vi "Wave-Read EPL Chunk.vi"(0 "Wave File":path, 11 "error in (no error)":errorcluster) -> (8 "EPL Variables":T1[](array[typedef]), 15 "error out":errorcluster)   [LabVIEW 2020]
uses:
  Wave-EPL Chunk Variable.ctl
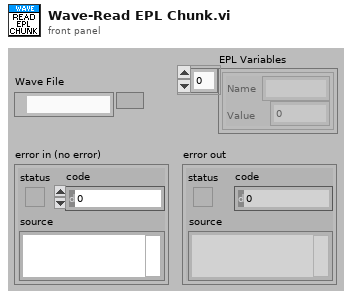
[diagram p1: front panel]
types:
  T1 = typedef "Wave-EPL Chunk Variable.ctl" = cluster{"Name":string, "Value":dbl}
  T2 = typedef "Wave-Chunk Info.ctl" = cluster{"ID":string, "Size":u32}
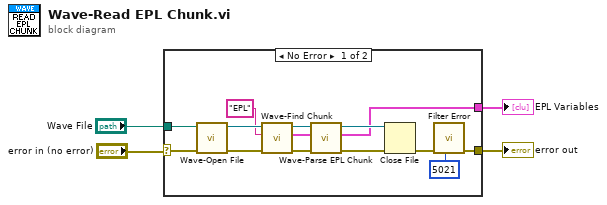
[diagram p0: block diagram]
diagram:
  n1 = case shown="No Error" "error in (no error)" {
    selector: "error in (no error)" -> [w16 w19]
    tunnel: [w6 w19] -> w3
    tunnel: "Wave File" -> [w18 _]
    tunnel: [w7 _] -> w1
    frame No Error {
      n2 = call "Wave-Open File.vi"("error in (no error)"=w16, "Path"=w18) -> ("error out"=w17:errorcluster, "refnum out"=w14:refnum<file>)  [unwired: 8 in]
      n3 = call "Wave-Find Chunk.vi"("error in (no error)"=w17, "Chunk ID"="EPL", "Refnum"=w14) -> ("error out"=w12:errorcluster, "chunk info"=w10:T2, "refnum out"=w11:refnum<file>)  [unwired: 6 in]
      n4 = call "Wave-Parse EPL Chunk.vi"("error in (no error)"=w12, "chunk info"=w10, "refnum"=w11) -> ("error out"=w9:errorcluster, "EPL Variables"=w7:T1[], "refnum out"=w8:refnum<file>)  [unwired: 6 in]
      n5 = Close File(refnum=w8, error in=w9) -> (error out=w15:errorcluster)  [unwired: 1 out]
      n6 = call "Filter Error.vi"("error in (no error)"=w15, "code to ignore"=5021) -> ("error out"=w6:errorcluster)  [unwired: 9 in]
    }
    frame Error {
    }
  }
  "error out" <- w3
  "EPL Variables" <- w1
